vi "updateDB.vi"(6 "First":bool, 8 "DBname":string, 9 "Data Write":i32[](array[numeric]), 10 "Write?":bool, 11 "COM PORT":refnum<visa-resource-name>) -> (0 "Written!":bool, 3 "DBarray":dbl[][](array[numeric]), 4 "First 2":bool)   [LabVIEW 2024]
panel:
  out "Written!":bool
  out "RX_DATA":i32[](array[numeric])
  out "DB_data":dbl[](array[numeric])
  out "i":i32
  out "IDs No":dbl
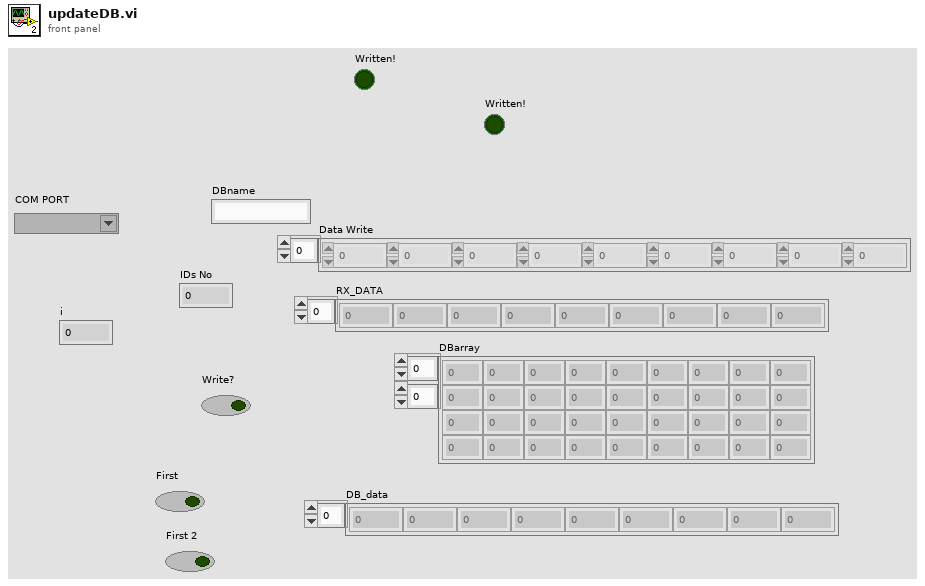
[diagram p1: front panel]
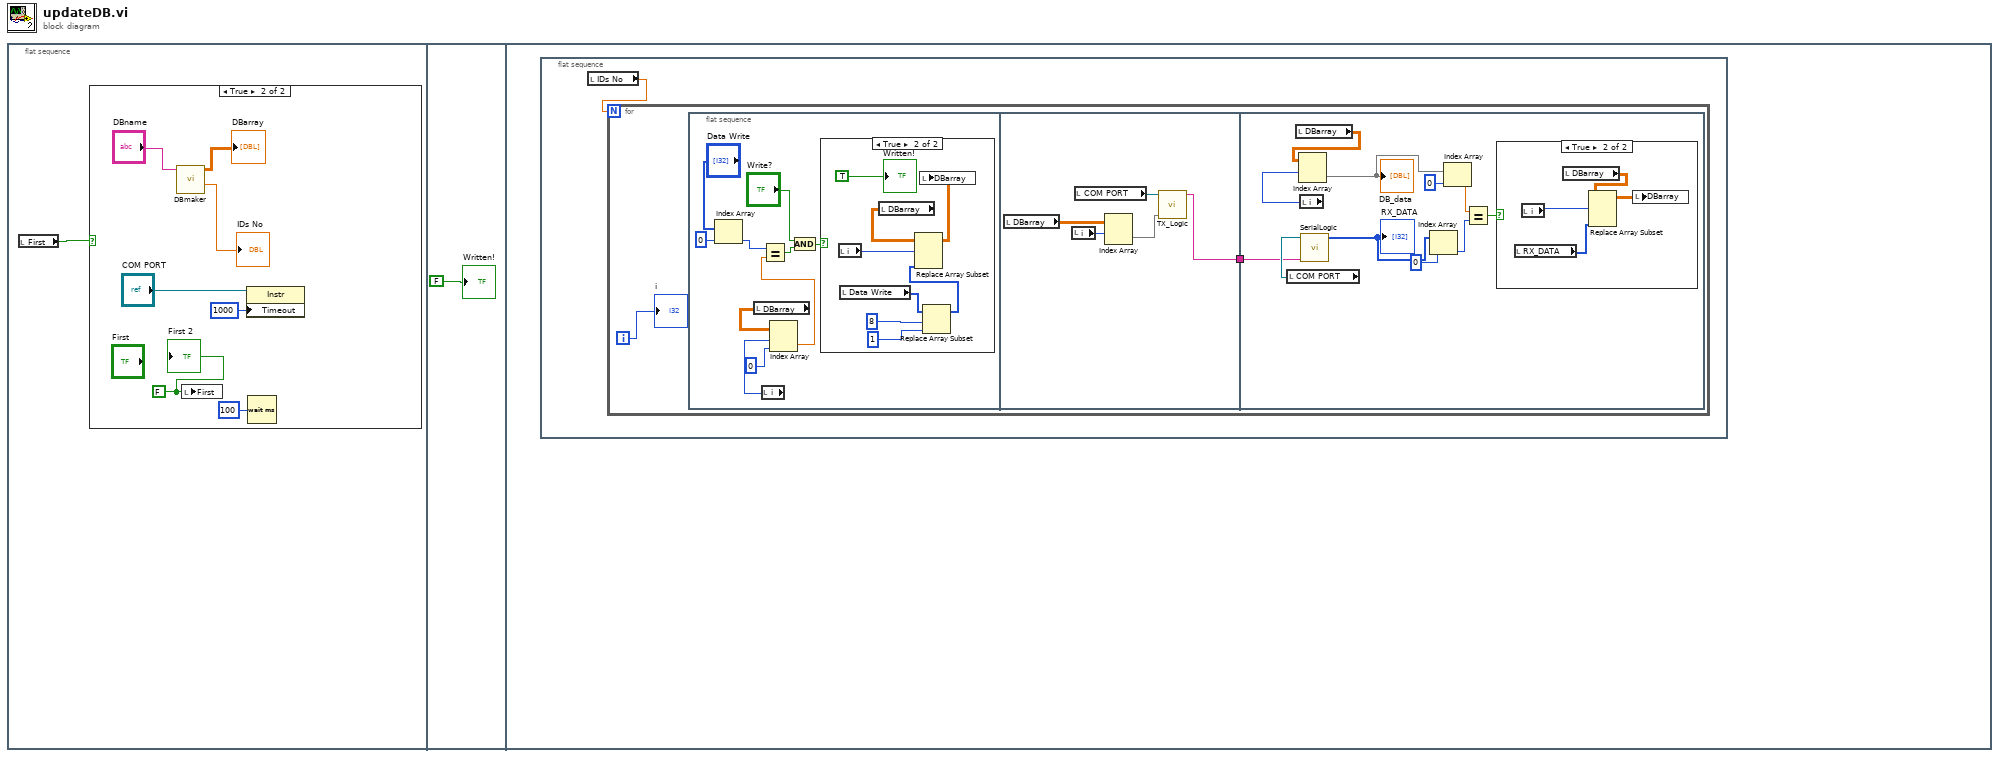
[diagram p0: block diagram]
diagram:
  n1 = flat-sequence {
    frame #0 {
      n2 = local read "First"() -> (w1:bool)
      n3 = case shown="True" w1 {
        frame False {
        }
        frame True {
          w5 = FALSE ("First")
          n4 = call "DBmaker.vi"("DBname"="DBname") -> ("IDs No"=→"IDs No":dbl, "DBarray"=→"DBarray":dbl[][])  [unwired: 7 in]
          n5 = local write "First"(w5) -> ()
          n6 = property class="Instr"(reference="COM PORT", "Timeout"=u32 1000 ("General Settings:Timeout Value")) -> ()  [unwired: 1 in, 2 out]
          n7 = Wait (ms)(milliseconds to wait=u32 100) -> ()  [unwired: 1 out]
          "First 2" <- w5
        }
      }
    }
    frame #1 {
      "Written!" <- FALSE ("Written!")
    }
    frame #2 {
      n8 = flat-sequence {
        frame #0 {
          n9 = local read "IDs No"() -> (w10:dbl)
          n10 = for {
            N: w10 -> [_]
            i -> [w12]
            n11 = flat-sequence {
              tunnel: [w31] -> w11
              tunnel: w11 -> [w36]
              frame #0 {
                n12 = Index Array(array="Data Write", index=0) -> (element=w13:i32)
                n13 = local read "DBarray"() -> (w20:dbl[][])
                n14 = local read "i"() -> (w19:i32)
                n15 = Index Array(array=w20, index (row)=w19, index (col)=0 ("disabled index (col)")) -> (element=w16:dbl)
                n16 = Equal?(x=w13, y=w16) -> (x = y?=w17:bool)
                n17 = And(x="Write?", y=w17) -> (x .and. y?=w22:bool)
                n18 = case shown="True" w22 {
                  frame False {
                  }
                  frame True {
                    n19 = local read "i"() -> (w28:i32)
                    n20 = local read "Data Write"() -> (w27:i32[])
                    n21 = local read "DBarray"() -> (w30:dbl[][])
                    n22 = Replace Array Subset(array=w27, new element=1 ("new element/subarray"), index=8) -> (w26:i32[])
                    n23 = Replace Array Subset(array=w30, new element=w26, index (row)=w28) -> (w29:dbl[][])  [unwired: 1 in]
                    n24 = local write "DBarray"(w29) -> ()
                    "Written!" <- TRUE ("Written!")
                  }
                }
              }
              frame #1 {
                n25 = local read "DBarray"() -> (w35:dbl[][])
                n26 = local read "i"() -> (w34:i32)
                n27 = local read "COM PORT"() -> (w33:refnum<visa-resource-name>)
                n28 = Index Array(array=w35, index (row)=w34) -> (element=w32:dbl[])  [unwired: 1 in]
                n29 = call "TX_Logic.vi"("initialized array 2"=w32, "VISA resource name"=w33) -> ("read buffer"=w31:string)  [unwired: 7 in]
              }
              frame #2 {
                n30 = local read "COM PORT"() -> (w44:refnum<visa-resource-name>)
                n31 = local read "DBarray"() -> (w46:dbl[][])
                n32 = local read "i"() -> (w45:i32)
                n33 = Index Array(array=w46, index (row)=w45) -> (element=w42:dbl[])  [unwired: 1 in]
                "DB_data" <- w42
                n34 = call "SerialLogic.vi"("read buffer"=w36, "COM PORT"=w44) -> ("RX_DATA"=w38:i32[])  [unwired: 9 in]
                "RX_DATA" <- w38
                n35 = Index Array(array=w38, index=0) -> (element=w39:i32)
                n36 = Index Array(array=w42, index=0) -> (element=w40:dbl)
                n37 = Equal?(x=w40, y=w39) -> (x = y?=w43:bool)
                n38 = case shown="True" w43 {
                  frame False {
                  }
                  frame True {
                    n39 = local read "RX_DATA"() -> (w47:i32[])
                    n40 = local read "i"() -> (w49:i32)
                    n41 = local read "DBarray"() -> (w50:dbl[][])
                    n42 = Replace Array Subset(array=w50, new element=w47, index (row)=w49) -> (w48:dbl[][])  [unwired: 1 in]
                    n43 = local write "DBarray"(w48) -> ()
                  }
                }
              }
            }
            "i" <- w12
          }
        }
      }
    }
  }
